vi "One Button PoP Up.vi"(7 "Message In":string) -> ()   [LabVIEW 2016, in "User Interface.lvlib"]
uses:
  User Interface.lvlib
panel:
  in  "OK Button":bool
  out "Msg Out":string
  out "Time":string="Sat  8/3/2019  8:10:44 PM"
  out "error out":errorcluster
  in  "error in (no error)":errorcluster
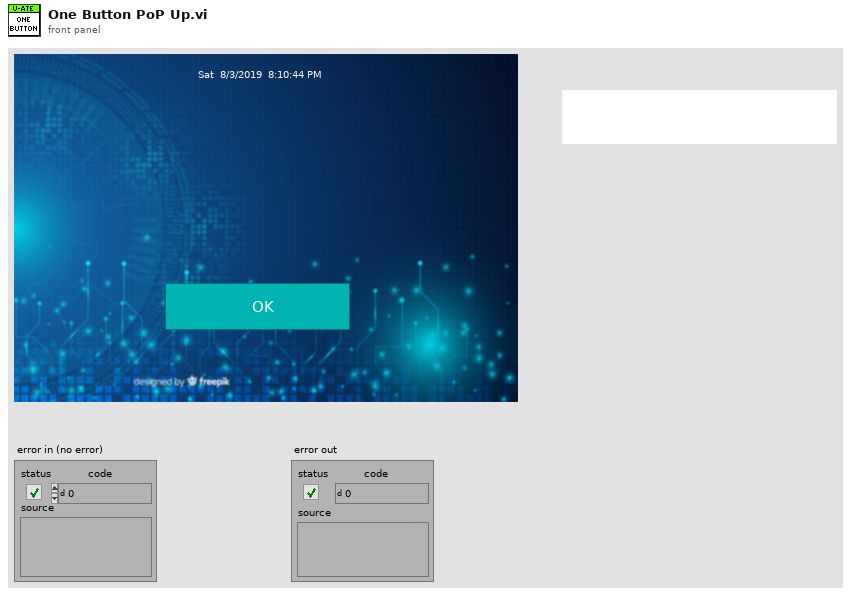
[diagram p1: front panel]
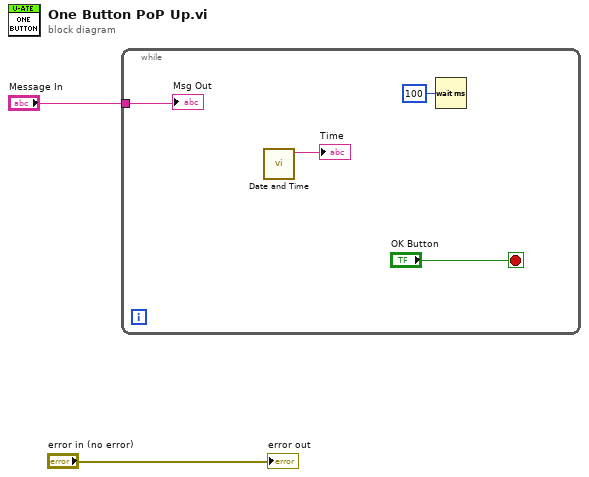
[diagram p0: block diagram]
diagram:
  n1 = while {
    tunnel: "Message In" -> [w4]
    stop <- "OK Button" stop-if-true
    n2 = call "Date and Time.vi"() -> ("Current Time"=→"Time":string)  [unwired: 11 in]
    n3 = Wait (ms)(milliseconds to wait=u32 100) -> ()  [unwired: 1 out]
    "Msg Out" <- w4
  }
  "error out" <- "error in (no error)"
